vi "ImageGlobal.vi"() -> ()   [LabVIEW 2017]
panel:
  out "Image":T1(plugin-control)
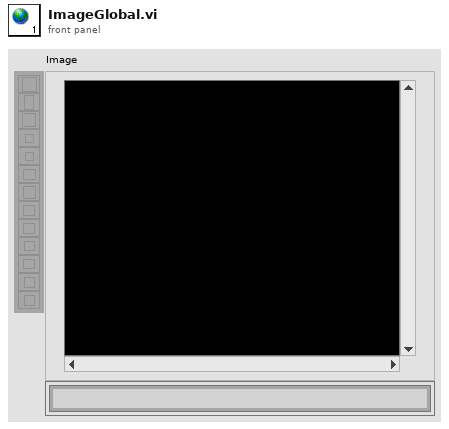
[diagram p1: front panel]
types:
  T1 = typedef "IMAQ Image.ctl" = refnum<image>
diagram:
